vi "checkResistance.vi"(7 "Thermistor Resistance ratio\n R_T(T1) / R_T(T1+1)":dbl=0.96, 8 "Current Resistance":dbl, 9 "Set Temperature":dbl, 10 "Calibrated Temperature":dbl, 11 "Calibrated Resistance":dbl) -> (2 "Current Temperature":dbl, 3 "Turn Voltage On?":bool)   [LabVIEW 2013]
panel:
  out "ratio":dbl
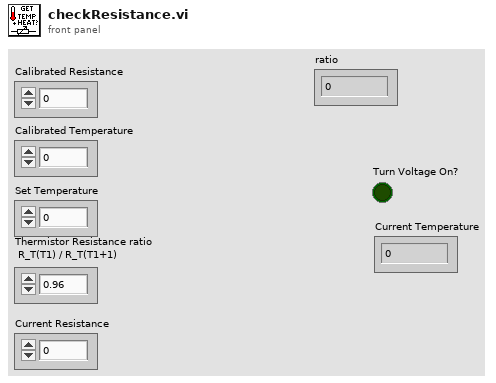
[diagram p1: front panel]
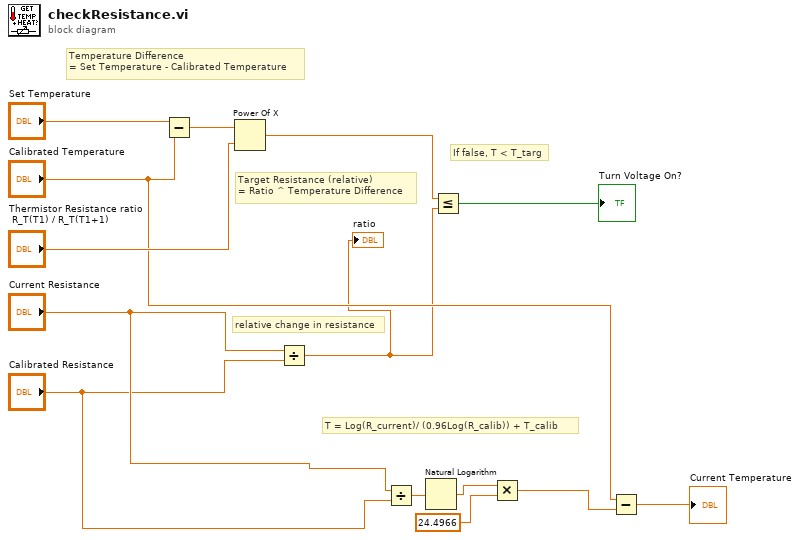
[diagram p0: block diagram]
diagram:
  # "T = Log(R_current)/ (0.96Log(R_calib)) + T_calib"
  # "If false, T < T_targ"
  # "relative change in resistance"
  # "Target Resistance (relative)\n= Ratio ^ Temperature Difference"
  # "Temperature Difference\n= Set Temperature - Calibrated Temperature"
  n1 = Subtract(x="Set Temperature", y="Calibrated Temperature") -> (x-y=w13:dbl)
  n2 = Power Of X(1:"Thermistor Resistance ratio\n R_T(T1) / R_T(T1+1)", 2:w13) -> (0:w12:dbl)
  n3 = Divide(x="Current Resistance", y="Calibrated Resistance") -> (x/y=w7:dbl)
  "ratio" <- w7
  n4 = Divide(x="Current Resistance", y="Calibrated Resistance") -> (x/y=w4:dbl)
  n5 = Natural Logarithm(1:w4) -> (0:w3:dbl)
  n6 = Less Or Equal?(x=w12, y=w7) -> (x <= y?=→"Turn Voltage On?":bool)
  n7 = Multiply(x=w3, y=24.4966) -> (x*y=w1:dbl)
  n8 = Subtract(x="Calibrated Temperature", y=w1) -> (x-y=→"Current Temperature":dbl)
